vi "Get ClassItems from ProjectItem.vi"(8 "error in (no error)":errorcluster, 11 "ProjectItem in":refnum<vi>) -> (0 "error out":errorcluster, 1 "Class Item Names":string[](array[string]), 2 "Class Items":refnum<vi>[](array[refnum]), 3 "ProjectItem out":refnum<vi>)   [LabVIEW 2019, in "VI Scripting Tools.lvlib"]
uses:
  VI Scripting Tools.lvlib
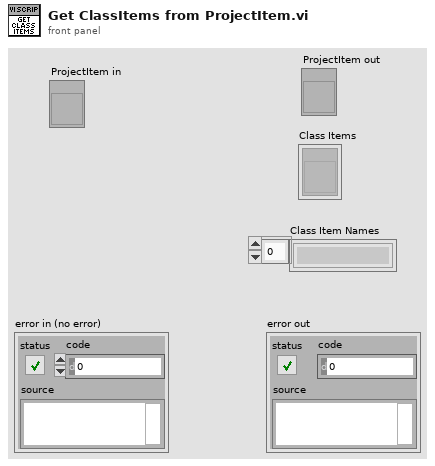
[diagram p1: front panel]
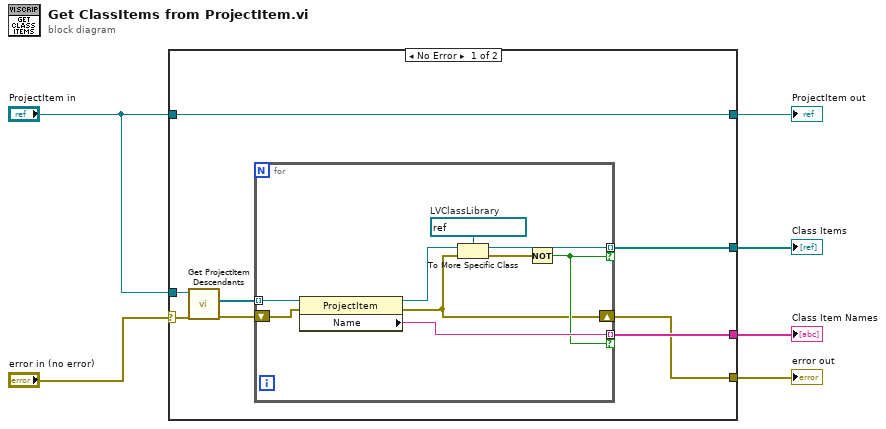
[diagram p0: block diagram]
diagram:
  n1 = case shown="No Error" "error in (no error)" {
    selector: "error in (no error)" -> [w7 w24]
    tunnel: "ProjectItem in" -> [w14 _]
    tunnel: [w12 _] -> w6
    tunnel: [w10 _] -> w5
    tunnel: [w9 w24] -> w4
    tunnel: "ProjectItem in" -> [w8 w25]
    tunnel: [w8 w25] -> w2
    frame No Error {
      n2 = call "Get ProjectItem Descendants.vi"("error in (no error)"=w7, "ProjectItem in"=w14) -> ("error out"=w13:errorcluster, "All Descendents"=w11:refnum<vi>[])  [unwired: 7 in, 1 out]
      n3 = for {
        tunnel: w11 -> [w23] mode=indexing
        tunnel: [w22] -> w12 mode=indexing if=w17
        tunnel: [w18] -> w10 mode=indexing if=w17
        shift-right: [w15] -> w9
        shift-left: w13 -> [w16]
        w21 = refnum<vi> refnum  # LVClassLibrary
        n4 = property class="ProjectItem"(reference=w23, error in=w16) -> (reference out=w19:refnum<vi>, error out=w15:errorcluster, "Name"=w22:string)
        n5 = To More Specific Class(target class=w21, reference=w19, error in=w15) -> (specific class reference=w18:refnum<vi>, error out=w20:errorcluster)
        n6 = Not(x=w20) -> (.not. x?=w17:bool)
      }
    }
    frame Error {
    }
  }
  "Class Item Names" <- w6
  "Class Items" <- w5
  "ProjectItem out" <- w2
  "error out" <- w4
